vi "process-percent.vi"() -> ()   [LabVIEW 2013]
panel:
  in  "字符串":string="正在载入中.......请稍等 ~"
  out "水平刻度条":dbl(slide) scale=0.0..100.0
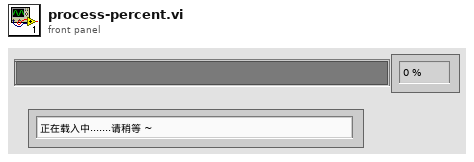
[diagram p1: front panel]
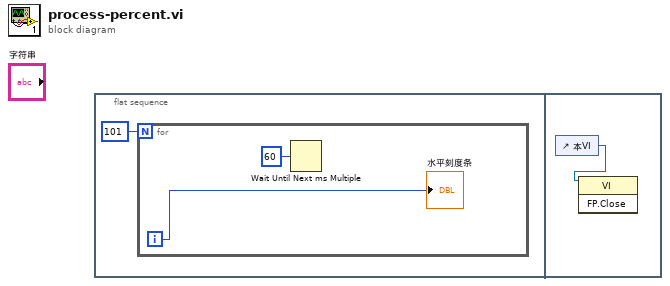
[diagram p0: block diagram]
diagram:
  n1 = flat-sequence {
    frame #0 {
      n2 = for {
        N: 101 -> [_]
        i -> [w3]
        n3 = Wait Until Next ms Multiple(millisecond multiple=u32 60 ("毫秒倍数")) -> ()  [unwired: 1 out]
        "水平刻度条" <- w3
      }
    }
    frame #1 {
      n4 = control-ref of="本VI"() -> (w4:refnum<vi>)
      n5 = invoke class="VI" method="FP.Close"(reference=w4) -> ()  [unwired: 2 in, 3 out]
    }
  }
